vi "emi_Split string.vi"(0 "String":string, 7 "Split index(0)":i32, 11 "error in (no error)":errorcluster) -> (4 "Substring Start":string, 8 "Substring End":string, 15 "error out":errorcluster)   [LabVIEW 2010]
doc: "Splits a string in two.\ns\nIf index is 0 or less. Substring End will contain the whole string, and Substring Start will be empty.\nIf index is equal or larger then the lengt of the string, Substring Start will contain the whole string, and Substring End will be empty.\n\nOn Error: No action\n\nFor large string(more then 10kbyte) it is nost recomended to use this vi, but do the splitting directly. This is to avoid the copying that may happen with passing strings through cases and VI \"wals\".\n\nSub routine for throughput"
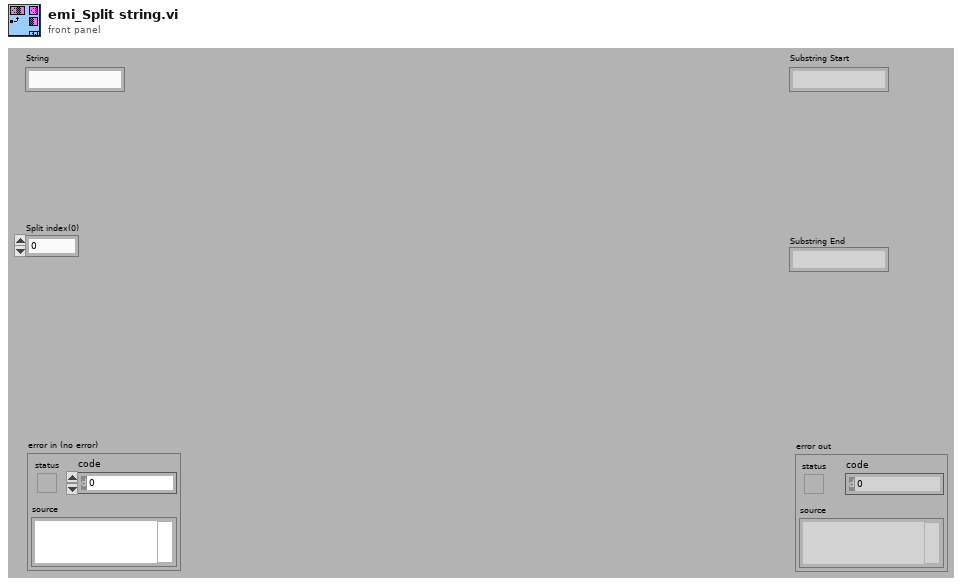
[diagram p1: front panel]
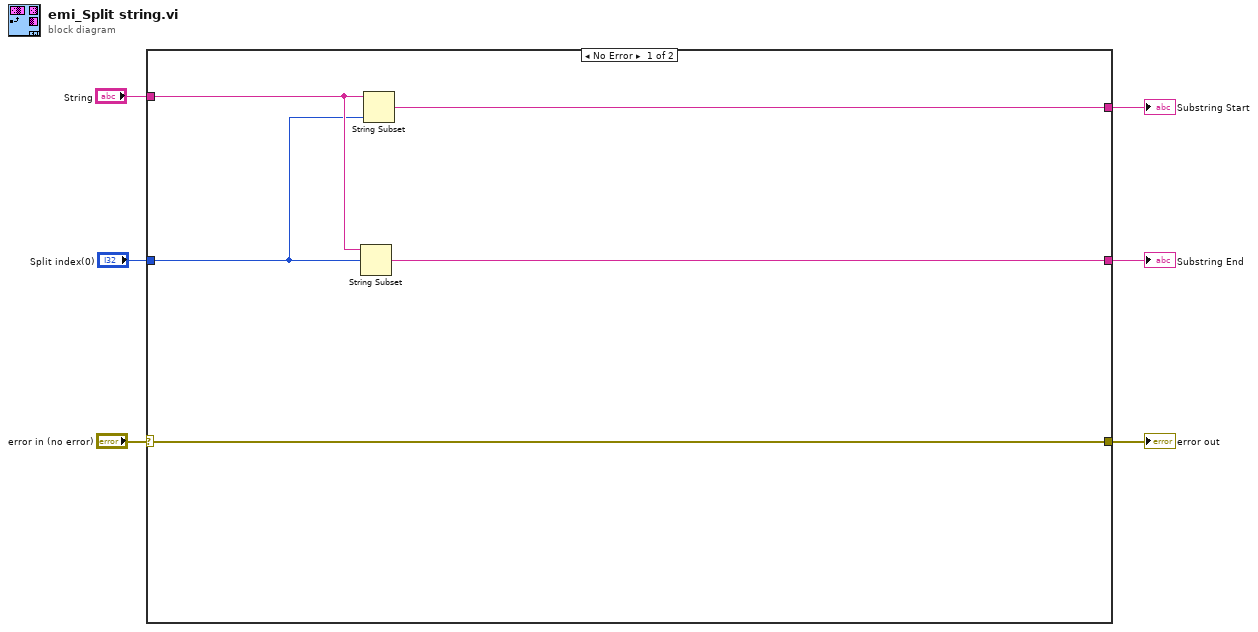
[diagram p0: block diagram]
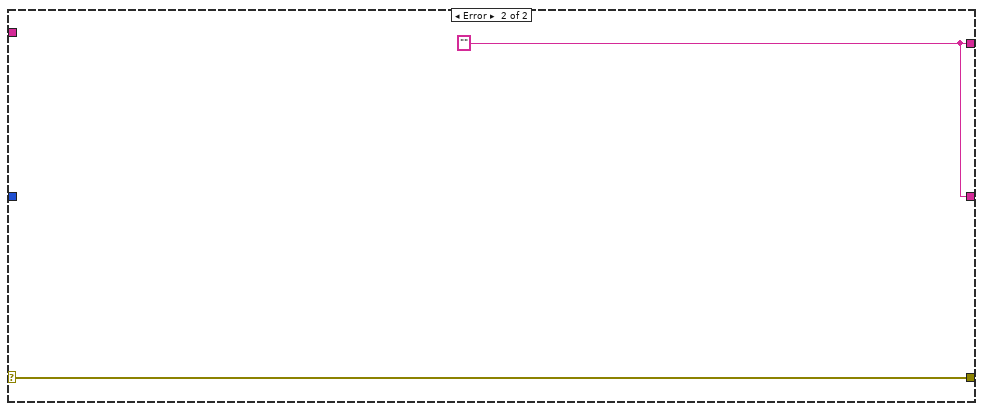
[diagram p2: hidden frame]
diagram:
  n1 = case shown="No Error" "error in (no error)" {
    selector: "error in (no error)" -> [w11 w13]
    tunnel: [w11 w13] -> w5
    tunnel: "String" -> [w10 _]
    tunnel: "Split index(0)" -> [w9 _]
    tunnel: [w8 w12] -> w2
    tunnel: [w7 w12] -> w1
    frame No Error {
      n2 = String Subset(string=w10, offset (0)=w9) -> (substring=w7:string)  [unwired: 1 in]
      n3 = String Subset(string=w10, length (rest)=w9) -> (substring=w8:string)  [unwired: 1 in]
    }
    frame Error {
      w12 = "" ("String")
    }
  }
  "error out" <- w5
  "Substring End" <- w1
  "Substring Start" <- w2
